vi "FixedRampPaths_calc.vi"(4 "#Points":u32[](array[numeric])=[0, 30, 1, 20] step=1, 6 "RampSelect":bool[](array[boolean]), 7 "File Path Para Array out":T1[](array[typedef])) -> (3 "Path array":path[](array[path]))   [LabVIEW 2020]
uses:
  Globals and TypeDefs/Type Definitions.llb/FilePathParameter.ctt
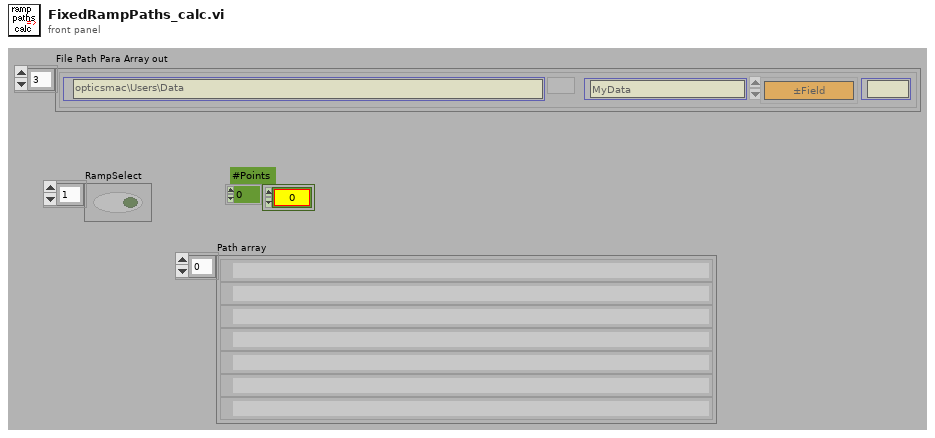
[diagram p1: front panel]
types:
  T1 = typedef "FilePathParameter.ctt" = cluster{"Filename Prefix":string, "Extension":enum16{"none", "\".001\",\".002\", ...", "001 (No dot)", "±Field", "pField nField", "Temperature", "Wavelength", "T(K)±H(T)", "(nm)T(K)±H(T)", "User Defined"}, "Suffix":string, "Current Path":path}
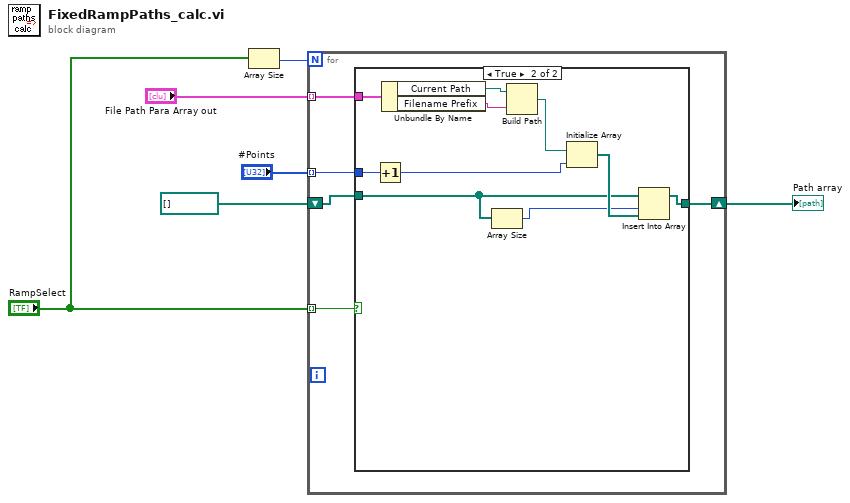
[diagram p0: block diagram]
diagram:
  n1 = Array Size(array="RampSelect") -> (size(s)=w4:i32)
  n2 = for {
    N: w4 -> [_]
    tunnel: "RampSelect" -> [w11] mode=indexing
    tunnel: "#Points" -> [w10] mode=indexing
    tunnel: "File Path Para Array out" -> [w9] mode=indexing
    shift-right: [w7] -> w1
    shift-left: path[] [] ("initialized array") -> [w8]
    n3 = case shown="True" w11 {
      tunnel: w10 -> [_ w22]
      tunnel: w9 -> [_ w21]
      tunnel: w8 -> [w12 w15]
      tunnel: [w12 w13] -> w7
      frame False {
      }
      frame True {
        n4 = Increment(x=w22) -> (x+1=w17:u32)
        n5 = Unbundle By Name(w21) -> ("Current Path"=w20:path, "Filename Prefix"=w19:string)
        n6 = Array Size(array=w15) -> (size(s)=w14:i32)
        n7 = Build Path(base path=w20, name or relative path=w19) -> (appended path=w18:path)
        n8 = Initialize Array(w18, w17) -> (w16:path[])
        n9 = Insert Into Array(array=w15, index=w14, new element=w16) -> (w13:path[])
      }
    }
  }
  "Path array" <- w1
